vi "1D Fit Max Relative Residual.vi"(8 "error in (no error)":errorcluster, 10 "Residual Plot":cluster{"X Array":dbl[], "Y Array":dbl[]}, 11 "Plot":cluster{"X Array":dbl[], "Y Array":dbl[]}) -> (0 "error out":errorcluster, 1 "Max Relative Residual":dbl, 2 "Residual Plot (dup)":cluster{"X Array":dbl[], "Y Array":dbl[]})   [LabVIEW 2021, in "Fits.lvlib"]
doc: "Computes the Maximum Relative Residual of a fit, defined as the max absolute residual divided by the plot value.\n\nNaN values are ignored."
uses:
  Fits.lvlib
panel:
  # "see the License on the block diagram (Ctrl+E or Window:Show Block Diagram)"
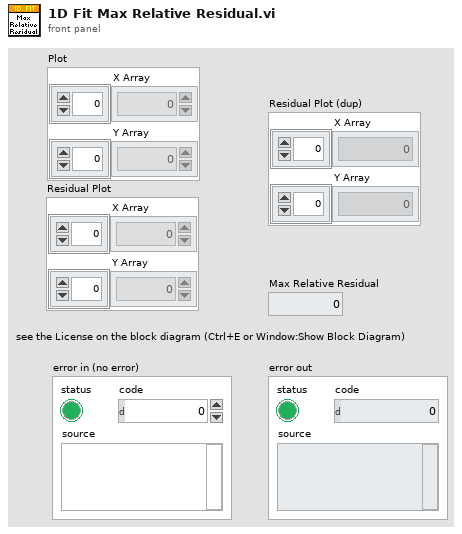
[diagram p1: front panel]
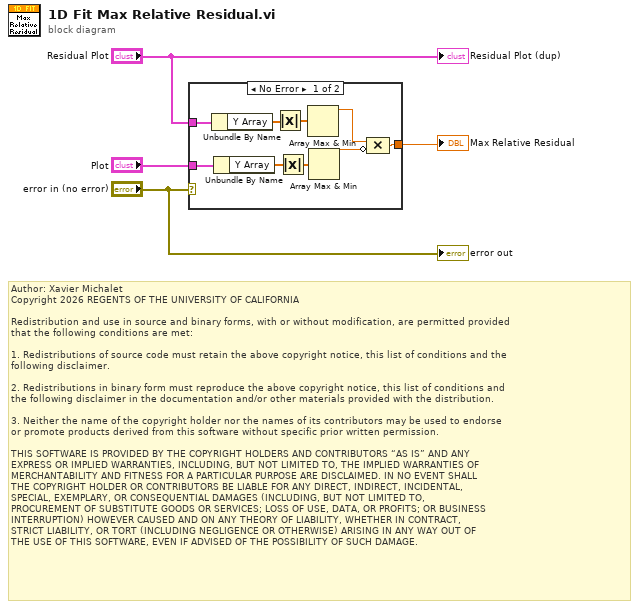
[diagram p0: block diagram]
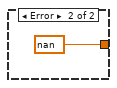
[diagram p2: hidden frame]
diagram:
  # "Author: Xavier Michalet\nCopyright 2026 REGENTS OF THE UNIVERSITY OF CALIFORNIA\n\nRedistribution and use in source and binary forms, with or without modification, are permitted provided\nthat the following conditions are met:\n\n1. Redistributions of source code must retain the above copyright notice, this list of conditions and the\nfollowing disclaimer.\n\n2. Redistributions in binary form must reproduce the above copyright notice, this list of conditions and\nthe following disclaimer in the documentation and/or other materials provided with the distribution.\n\n3. Neither the name of the copyright holder nor the names of its contributors may be used to endorse \nor promote products derived from this software without specific prior written permission.\n\nTHIS SOFTWARE IS PROVIDED BY THE COPYRIGHT HOLDERS AND CONTRIBUTORS “AS IS” AND ANY \nEXPRESS OR IMPLIED WARRANTIES, INCLUDING, BUT NOT LIMITED TO, THE IMPLIED WARRANTIES OF\nMERCHANTABILITY AND FITNESS FOR A PARTICULAR PURPOSE ARE DISCLAIMED. IN NO EVENT SHALL\nTHE COPYRIGHT HOLDER OR CONTRIBUTORS BE LIABLE FOR ANY DIRECT, INDIRECT, INCIDENTAL, \nSPECIAL, EXEMPLARY, OR CONSEQUENTIAL DAMAGES (INCLUDING, BUT NOT LIMITED TO, \nPROCUREMENT OF SUBSTITUTE GOODS OR SERVICES; LOSS OF USE, DATA, OR PROFITS; OR BUSINESS\nINTERRUPTION) HOWEVER CAUSED AND ON ANY THEORY OF LIABILITY, WHETHER IN CONTRACT, \nSTRICT LIABILITY, OR TORT (INCLUDING NEGLIGENCE OR OTHERWISE) ARISING IN ANY WAY OUT OF\nTHE USE OF THIS SOFTWARE, EVEN IF ADVISED OF THE POSSIBILITY OF SUCH DAMAGE."
  n1 = case shown="No Error" "error in (no error)" {
    tunnel: "Residual Plot" -> [w13 _]
    tunnel: "Plot" -> [w12 _]
    tunnel: [w5 nan] -> w1
    frame No Error {
      n2 = Unbundle By Name(w13) -> ("Y Array"=w11:dbl[])
      n3 = Unbundle By Name(w12) -> ("Y Array"=w10:dbl[])
      n4 = Absolute Value(x=w11) -> (abs(x)=w9:dbl[])
      n5 = Absolute Value(x=w10) -> (abs(x)=w8:dbl[])
      n6 = Array Max & Min(array=w9) -> (max value=w7:dbl)  [unwired: 3 out]
      n7 = Array Max & Min(array=w8) -> (max value=w6:dbl)  [unwired: 3 out]
      n8 = Compound Arithmetic op=MULTIPLY(w7, invert w6) -> (w5:dbl)
    }
    frame Error {
    }
  }
  "Max Relative Residual" <- w1
  "error out" <- "error in (no error)"
  "Residual Plot (dup)" <- "Residual Plot"
